vi "Baby Demo.vi"() -> ()   [LabVIEW 2009]
uses:
  Baby/Baby.lvclass
  ISleepable/ISleepable.lvclass
  Baby/ISleepableBaby/ISleepableBaby.lvclass
  CellPhone/ISleepableCellPhone/ISleepableCellPhone.lvclass
  Source/Interfaceable Class/Interfaceable.lvclass
panel:
  out "results":bool[](array[boolean])
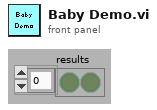
[diagram p1: front panel]
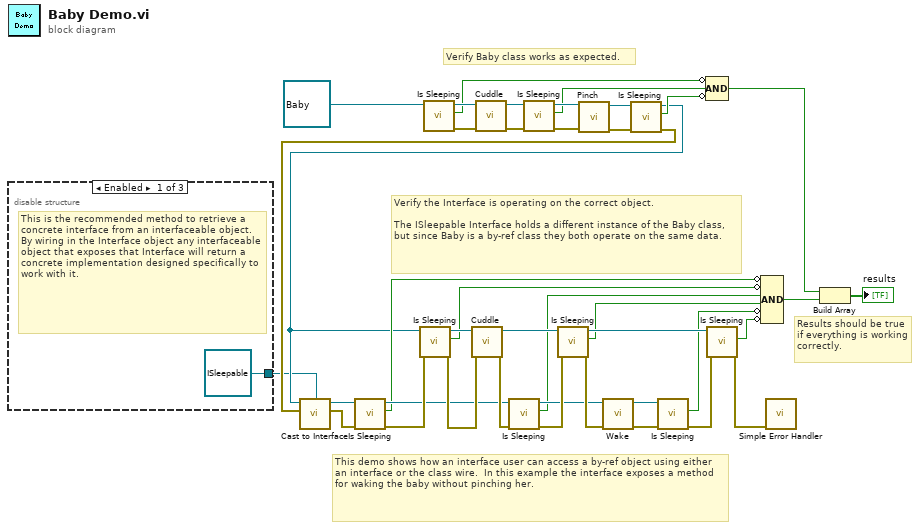
[diagram p0: block diagram]
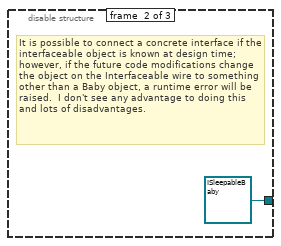
[diagram p2: hidden frame]
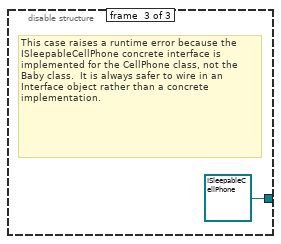
[diagram p3: hidden frame]
diagram:
  # "This demo shows how an interface user can access a by-ref object using either an interface or the class wire.  In this example the interface exposes a method for waking the baby without pinching her."
  # "Results should be true if everything is working correctly."
  # "Verify the Interface is operating on the correct object.\n\nThe ISleepable Interface holds a different instance of the Baby class, but since Baby is a by-ref class they both operate on the same data."
  # "Verify Baby class works as expected."
  n1 = disable-structure shown="Enabled" {
    disable-tunnel: [refnum<class "ISleepable.lvclass"> refnum ("ISleepable") refnum<class "ISleepableBaby.lvclass"> refnum ("ISleepableBaby.lvclass") refnum<class "ISleepableCellPhone.lvclass"> refnum ("CellPhone ISleepable")] -> w1
    frame #0 {
      # "This is the recommended method to retrieve a concrete interface from an interfaceable object.  By wiring in the Interface object any interfaceable object that exposes that Interface will return a concrete implementation designed specifically to work with it."
    }
    frame #1 {
      # "It is possible to connect a concrete interface if the interfaceable object is known at design time; however, if the future code modifications change the object on the Interfaceable wire to something other than a Baby object, a runtime error will be raised.  I don't see any advantage to doing this and lots of disadvantages."
    }
    frame #2 {
      # "This case raises a runtime error because the ISleepableCellPhone concrete interface is implemented for the CellPhone class, not the Baby class.  It is always safer to wire in an Interface object rather than a concrete implementation."
    }
  }
  n2 = call "Is Sleeping.vi"("Baby in"=refnum<class "Baby.lvclass"> refnum ("Baby")) -> ("error out"=w35:errorcluster, "IsSleeping"=w17:bool, "Baby out"=w37:refnum<class "Baby.lvclass">)  [unwired: 8 in]
  n3 = call "Cuddle.vi"("error in (no error)"=w35, "Baby in"=w37) -> ("error out"=w34:errorcluster, "Baby out"=w36:refnum<class "Baby.lvclass">)  [unwired: 8 in]
  n4 = call "Is Sleeping.vi"("error in (no error)"=w34, "Baby in"=w36) -> ("error out"=w32:errorcluster, "IsSleeping"=w16:bool, "Baby out"=w33:refnum<class "Baby.lvclass">)  [unwired: 7 in]
  n5 = call "Pinch.vi"("error in (no error)"=w32, "Baby in"=w33) -> ("error out"=w31:errorcluster, "Baby out"=w30:refnum<class "Baby.lvclass">)  [unwired: 8 in]
  n6 = call "Is Sleeping.vi"("error in (no error)"=w31, "Baby in"=w30) -> ("error out"=w4:errorcluster, "IsSleeping"=w15:bool, "Baby out"=w2:refnum<class "Baby.lvclass">)  [unwired: 7 in]
  n7 = call "Cast to Interface.vi"("Target Interface"=w1, "Interfaceable Object"=w2, "error in (no error)"=w4) -> ("Concrete Interface"=w7:refnum<class "ISleepable.lvclass">, "error out"=w6:errorcluster)  [unwired: 5 in]
  n8 = call-dynamic "Is Sleeping.vi"("error in (no error)"=w6, "ISleepable in"=w7) -> ("error out"=w28:errorcluster, "IsSleeping"=w9:bool, "ISleepable out"=w26:refnum<class "ISleepable.lvclass">)  [unwired: 7 in]
  n9 = call "Is Sleeping.vi"("error in (no error)"=w28, "Baby in"=w2) -> ("error out"=w40:errorcluster, "IsSleeping"=w10:bool, "Baby out"=w18:refnum<class "Baby.lvclass">)  [unwired: 7 in]
  n10 = call "Cuddle.vi"("error in (no error)"=w40, "Baby in"=w18) -> ("error out"=w27:errorcluster, "Baby out"=w25:refnum<class "Baby.lvclass">)  [unwired: 8 in]
  n11 = call-dynamic "Is Sleeping.vi"("error in (no error)"=w27, "ISleepable in"=w26) -> ("error out"=w24:errorcluster, "IsSleeping"=w11:bool, "ISleepable out"=w23:refnum<class "ISleepable.lvclass">)  [unwired: 7 in]
  n12 = call "Is Sleeping.vi"("error in (no error)"=w24, "Baby in"=w25) -> ("error out"=w39:errorcluster, "IsSleeping"=w12:bool, "Baby out"=w19:refnum<class "Baby.lvclass">)  [unwired: 7 in]
  n13 = call-dynamic "Wake.vi"("error in (no error)"=w39, "ISleepable in"=w23) -> ("error out"=w21:errorcluster, "ISleepable out"=w22:refnum<class "ISleepable.lvclass">)  [unwired: 8 in]
  n14 = call-dynamic "Is Sleeping.vi"("error in (no error)"=w21, "ISleepable in"=w22) -> ("error out"=w20:errorcluster, "IsSleeping"=w13:bool)  [unwired: 7 in, 1 out]
  n15 = Compound Arithmetic op=AND(invert w17, w16, invert w15) -> (w3:bool)
  n16 = call "Is Sleeping.vi"("error in (no error)"=w20, "Baby in"=w19) -> ("error out"=w5:errorcluster, "IsSleeping"=w14:bool)  [unwired: 7 in, 1 out]
  n17 = Compound Arithmetic op=AND(invert w9, invert w10, w11, w12, invert w13, invert w14) -> (w8:bool)
  n18 = call <vilib>:"Simple Error Handler.vi"("error in (no error)"=w5) -> ()  [unwired: 4 in, 5 out]
  n19 = Build Array(w3, w8) -> (→"results":bool[])
